vi "Calibrate filter wheel.vi"(8 "Error In":errorcluster) -> (0 "error out":errorcluster, 1 "Rotation time (ms)":dbl, 2 "Enable Channel out":u8=11, 3 "Serial Port out":refnum<visa-resource-name>="COM3", 4 "No of points":i32, 5 "VISA resource name out":refnum<visa-resource-name>)   [LabVIEW 2016]
uses:
  <vilib>/MakerHub/LINX/Public/Peripherals/Digital/Digital Write 1 Chan.vi
  C:/Program Files (x86)/National Instruments/LabVIEW 2016/instr.lib/keithley_24xx/Keithley 24XX/Keithley 24XX.lvlib
panel:
  in  "Angle (degrees)":dbl=360.0
  in  "Clockwise?":bool=TRUE
  in  "Enable Channel":u8=11
  in  "Direction Channel":u8=8
  in  "Step Channel":u8=9
  in  "Serial Port":refnum<visa-resource-name>="COM6"
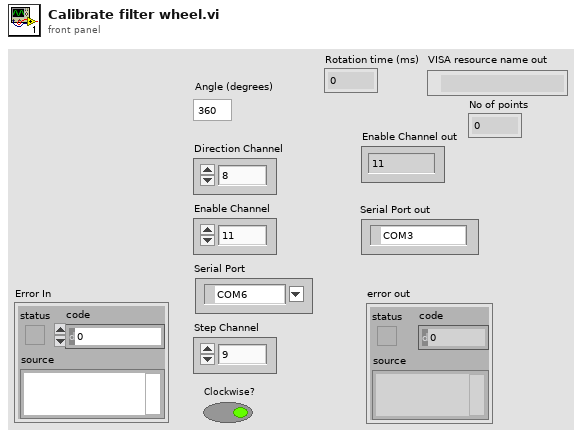
[diagram p1: front panel]
types:
  T1 = typedef "LMH-LINX.lvlib/LINX Ref.ctl" = cluster{"Platform":T2, "Interface":T3, "LINX Device Config":T4}
  T2 = typedef "LMH-LINX.lvlib/Platform.ctl" = enum16{"LINX", "myRIO"}
  T3 = typedef "LMH-LINX.lvlib/Interface.ctl" = enum16{"Serial", "TCP"}
  T4 = typedef "LMH-LINX.lvlib/Device.lvlib/LINX Device Config.ctl" = cluster{"Interface":T3, "COM Port":refnum<visa-resource-name>, "TCP Configuration":T5, "Device Family":u8, "Device ID":u8, "Device Name":string, "TCP Ref":refnum<k5>, "Channels":T6}
  T5 = typedef "LMH-LINX.lvlib/Device.lvlib/TCP Config.ctl" = cluster{"IP Address":string, "Port":u16}
  T6 = typedef "LMH-LINX.lvlib/Channels.ctl" = cluster{"DI":u8[], "DO":u8[], "AI":u8[], "AO":u8[], "PWM":u8[], "QE":u8[], "UART":u8[], "I2C 2":u8[], "SPI":u8[], "CAN":u8[], "Servo":u8[], "AI Ref (V)":dbl, "AO Ref (V)":dbl, "AO Resolution (Bits)":u8}
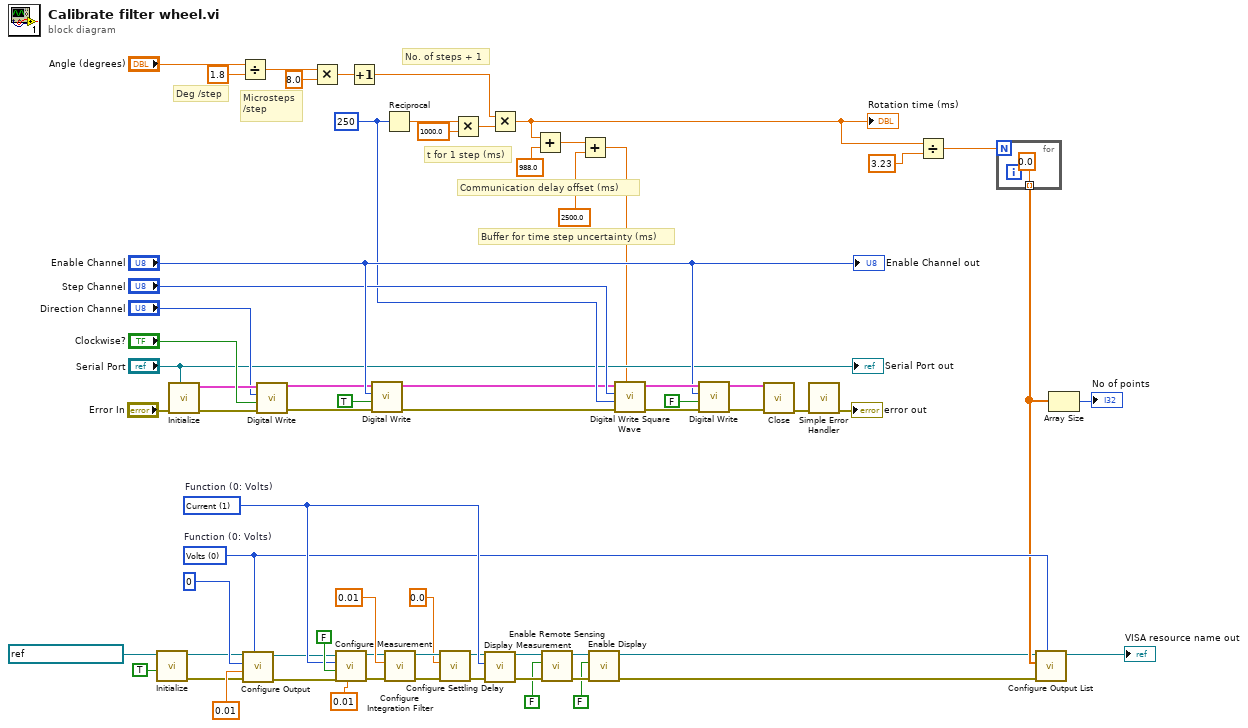
[diagram p0: block diagram]
diagram:
  w18 = u16 0 items=["Volts", "Current", "Resistance"]  # Function (0: Volts)
  w37 = u16 1 items=["Volts", "Current", "Resistance"]  # Function (0: Volts)
  w13 = u32 250 ("Frequency (Hz)")
  # "Buffer for time step uncertainty (ms)"
  # "Communication delay offset (ms)"
  # "t for 1 step (ms)"
  # "No. of steps + 1"
  # "Microsteps\n/step"
  # "Deg /step"
  n1 = call <vilib>:"Initialize.vi"("Reset (True)"=TRUE, "VISA resource name"=refnum<visa-resource-name> "GPIB0::24::INSTR") -> ("error out"=w21:errorcluster, "VISA resource name out"=w22:refnum<visa-resource-name>)  [unwired: 3 in, 5 out]
  n2 = call <vilib>:"Initialize.vi"("Serial Port"="Serial Port", "Error In"="Error In") -> ("Error Out"=w58:errorcluster, "LINX Ref"=w59:T1)  [unwired: 7 in, 1 out]
  n3 = Divide(x="Angle (degrees)", y=1.8) -> (x/y=w50:dbl)
  n4 = call "Configure Output.vi"("Source Mode  (0: Voltage)"=w18, "error in (no error)"=w21, "Compliance  Level (0.1)"=0.01 ("Compliance  Level"), "Output Level (0)"=0, "VISA resource name"=w22) -> ("error out"=w19:errorcluster, "VISA resource name out"=w20:refnum<visa-resource-name>)  [unwired: 5 in]
  n5 = call-poly <vilib>:"Digital Write.vi"("Error In"=w58, "Output Value"="Clockwise?", "DO Channel"="Direction Channel", "LINX Resource"=w59) -> ("Error Out"=w53:errorcluster, "LINX Resource"=w54:T1)  [unwired: 6 in]
  n6 = Multiply(x=w50, y=8.0) -> (x*y=w45:dbl)
  n7 = call "Configure Measurement.vi"("Manual Range (1.0)"=0.01, "error in (no error)"=w19, "Enable Auto Range (T:Enable)"=FALSE, "Function (0: Volts)"=w37, "VISA resource name"=w20) -> ("error out"=w32:errorcluster, "VISA resource name out"=w31:refnum<visa-resource-name>)  [unwired: 5 in]
  n8 = Increment(x=w45) -> (x+1=w44:dbl)
  n9 = call-poly <vilib>:"Digital Write.vi"("Error In"=w53, "Output Value"=TRUE ("LED Value"), "DO Channel"="Enable Channel", "LINX Resource"=w54) -> ("Error Out"=w10:errorcluster, "LINX Resource"=w11:T1)  [unwired: 6 in]
  n10 = Reciprocal(x=w13) -> (1/x=w48:dbl)
  n11 = call "Configure Integration Filter.vi"("error in (no error)"=w32, "Measurement Speed (1 PLC)"=0.01, "VISA resource name"=w31) -> ("error out"=w39:errorcluster, "VISA resource name out"=w38:refnum<visa-resource-name>)  [unwired: 7 in]
  n12 = call "Configure Settling Delay.vi"("error in (no error)"=w39, "Manual Settling Delay (0 sec)"=0.0, "VISA resource name"=w38) -> ("error out"=w36:errorcluster, "VISA resource name out"=w35:refnum<visa-resource-name>)  [unwired: 7 in]
  n13 = Multiply(x=w48, y=1000.0) -> (x*y=w46:dbl)
  n14 = call "Display Measurement.vi"("error in (no error)"=w36, "Displayed Measurement (0: Voltage)"=w37, "VISA resource name"=w35) -> ("error out"=w34:errorcluster, "VISA resource name out"=w33:refnum<visa-resource-name>)  [unwired: 7 in]
  n15 = Multiply(x=w44, y=w46) -> (x*y=w5:dbl)
  "Rotation time (ms)" <- w5
  n16 = Add(x=w5, y=988.0) -> (x+y=w4:dbl)
  n17 = call "Enable Remote Sensing.vi"("error in (no error)"=w34, "Enable Remote Sensing (T: Enable)"=FALSE, "VISA resource name"=w33) -> ("error out"=w29:errorcluster, "VISA resource name out"=w30:refnum<visa-resource-name>)  [unwired: 7 in]
  n18 = Add(x=w4, y=2500.0) -> (x+y=w3:dbl)
  n19 = call "Enable Display.vi"("error in (no error)"=w29, "Enable Display (T: Enable)"=FALSE ("Enable Output (T: Enable)"), "VISA resource name"=w30) -> ("error out"=w7:errorcluster, "VISA resource name out"=w8:refnum<visa-resource-name>)  [unwired: 7 in]
  n20 = call <vilib>:"Digital Write Square Wave.vi"("Duration (ms)"=w3, "Error In"=w10, "Frequency (Hz)"=w13, "Channel"="Step Channel", "LINX Resource"=w11) -> ("Error Out"=w65:errorcluster, "LINX Resource"=w66:T1)  [unwired: 5 in]
  n21 = call-poly <vilib>:"Digital Write.vi"("Error In"=w65, "Output Value"=FALSE ("LED Value"), "DO Channel"="Enable Channel", "LINX Resource"=w66) -> ("Error Out"=w62:errorcluster, "LINX Resource"=w63:T1)  [unwired: 6 in]
  n22 = call <vilib>:"Close.vi"("Error In"=w62, "LINX Resource"=w63) -> ("Error Out"=w68:errorcluster)  [unwired: 8 in, 1 out]
  n23 = call <vilib>:"Simple Error Handler.vi"("error in (no error)"=w68) -> ("error out"=→"error out":errorcluster)  [unwired: 4 in, 4 out]
  n24 = Divide(x=w5, y=3.23 ("Time step (ms)")) -> (x/y=w1:dbl)
  n25 = for {
    N: w1 -> [_]
    tunnel: [0.0 ("y")] -> w17 mode=indexing
  }
  n26 = call "Configure Output List.vi"("Source Mode  (0: Voltage)"=w18, "error in (no error)"=w7, "Output List"=w17, "VISA resource name"=w8) -> ("VISA resource name out"=→"VISA resource name out":refnum<visa-resource-name>)  [unwired: 6 in, 1 out]
  n27 = Array Size(array=w17) -> (size(s)=→"No of points":i32)
  "Serial Port out" <- "Serial Port"
  "Enable Channel out" <- "Enable Channel"
